vi "MPU_Stick_Queues_FGV.vi"(8 "error in (no error)":errorcluster, 11 "Initialize ?":bool) -> (0 "error out":errorcluster, 3 "MPU_Stick_Queues":T1)   [LabVIEW 2017]
uses:
  Controls/MPU_Stick_Queues.ctl
  Controls/MPU_Stick_Queue_Element.ctl
  Controls/MPU_Stick_Queue_Commands.ctl
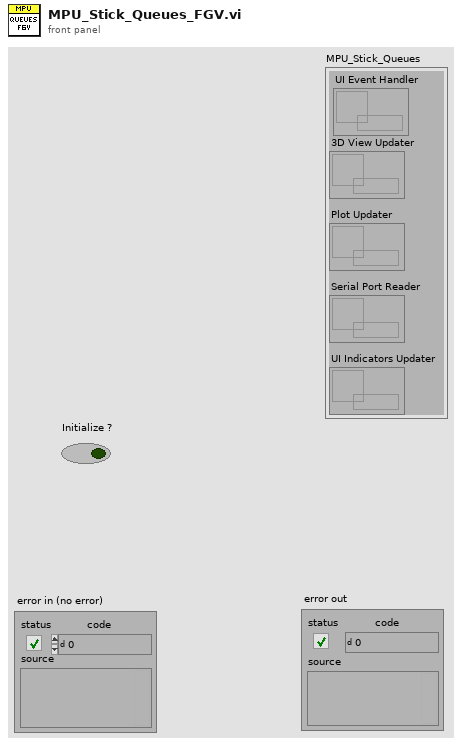
[diagram p1: front panel]
types:
  T1 = typedef "MPU_Stick_Queues.ctl" = cluster{"UI Event Handler":refnum<queue>, "3D View Updater":refnum<queue>, "Plot Updater":refnum<queue>, "Serial Port Reader":refnum<queue>, "UI Indicators Updater":refnum<queue>}
  T2 = typedef "MPU_Stick_Queue_Element.ctl" = cluster{"Data":variant, "Command":T3}
  T3 = typedef "MPU_Stick_Queue_Commands.ctl" = enum16{"UI_Event_Exit_Application_RQST", "UI_Event_Exit_Application_ACK", "UI_Event_Connect_Device_RQST", "UI_Event_Connect_Device_ACK", "UI_Event_Disconnect_Device_RQST", "UI_Event_Disconnect_Device_ACK", "UI_Event_Read_All_Configurations_RQST", "UI_Event_Read_All_Configurations_ACK", "UI_Event_Write_All_Configurations_RQST", "UI_Event_Write_All_Configurations_ACK", "UI_Event_Save_All_Configurations_RQST", "UI_Event_Save_All_Configurations_ACK", "UI_Event_Calibrate_IMU_Sensor_RQST", "UI_Event_Calibrate_IMU_Sensor_ACK", "UI_Event_MP_Reset_RQST", "UI_Event_MP_Reset_ACK", "UI_Event_Get_Config_RQST", "UI_Event_Get_Config_ACK", "UI_Event_Set_Config_RQST", "UI_Event_Set_Config_ACK", "Read_Serial_Port_Data_Pause", "Read_Serial_Port_Data_Continue", "Read_Serial_Port_Data_Exit", "Plotter_Exit", "Plotter_Update", "Plotter_Add_Channel", "Plotter_Remove_Channel", "3D Viewer Update", "3D Viewer Exit", "UI Indicators Update", "UI Indicators Exit"}
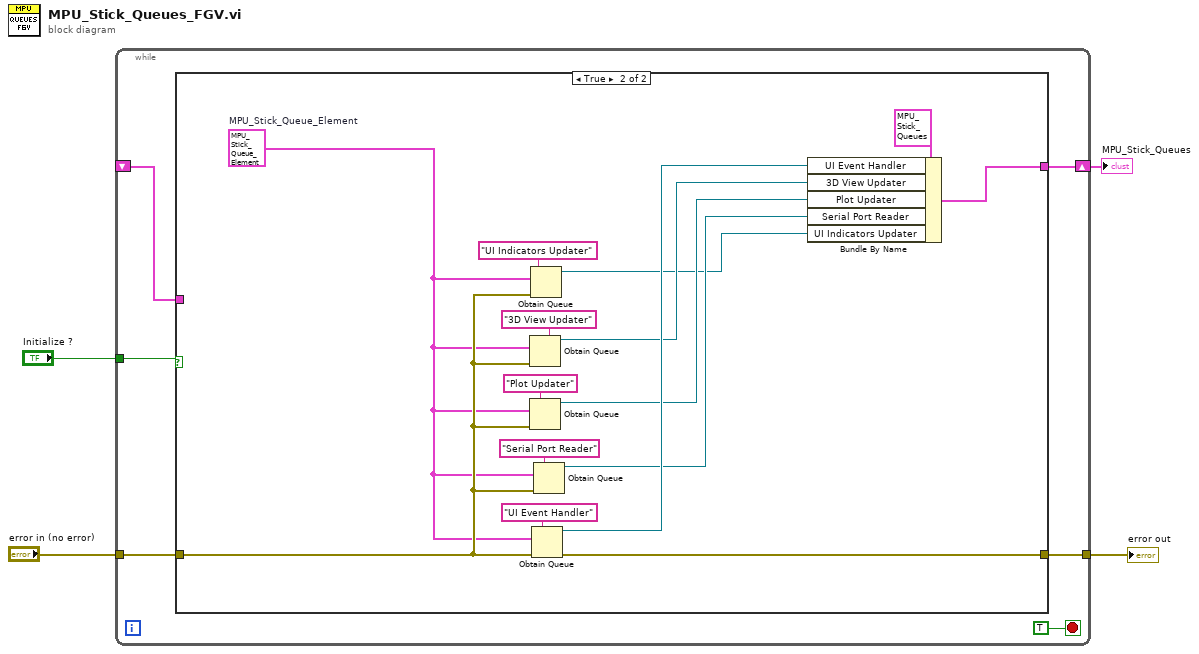
[diagram p0: block diagram]
diagram:
  n1 = while {
    tunnel: "error in (no error)" -> [w9]
    tunnel: [w8] -> w3
    shift-right: [w7] -> w2
    shift-left: _ -> [w6]
    tunnel: "Initialize ?" -> [w5]
    stop <- TRUE stop-if-true
    n2 = case shown="True" w5 {
      tunnel: w9 -> [w11 w15]
      tunnel: [w11 w27] -> w8
      tunnel: [w12 w23] -> w7
      tunnel: w6 -> [w12 _]
      frame False {
      }
      frame True {
        w13 = T2 {"Data"=variant, "Command"=enum."UI_Event_Exit_Application_RQST"}  # MPU_Stick_Queue_Element
        n3 = Obtain Queue(name (unnamed)="3D View Updater", element data type=w13, error in (no error)=w15) -> (queue out=w19:refnum<queue>)  [unwired: 2 in, 2 out]
        n4 = Obtain Queue(name (unnamed)="Plot Updater", element data type=w13, error in (no error)=w15) -> (queue out=w18:refnum<queue>)  [unwired: 2 in, 2 out]
        n5 = Obtain Queue(name (unnamed)="UI Indicators Updater", element data type=w13, error in (no error)=w15) -> (queue out=w14:refnum<queue>)  [unwired: 2 in, 2 out]
        n6 = Obtain Queue(name (unnamed)="UI Event Handler", element data type=w13, error in (no error)=w15) -> (queue out=w24:refnum<queue>, error out=w27:errorcluster)  [unwired: 2 in, 1 out]
        n7 = Obtain Queue(name (unnamed)="Serial Port Reader", element data type=w13, error in (no error)=w15) -> (queue out=w17:refnum<queue>)  [unwired: 2 in, 2 out]
        n8 = Bundle By Name(cluster=T1 {"UI Event Handler"=refnum, "3D View Updater"=refnum, "Plot Updater"=refnum, "Serial Port Reader"=refnum, "UI Indicators Updater"=refnum} ("MPU_Stick_Queues"), "UI Event Handler"=w24, "3D View Updater"=w19, "Plot Updater"=w18, "Serial Port Reader"=w17, "UI Indicators Updater"=w14) -> (w23:T1)
      }
    }
  }
  "error out" <- w3
  "MPU_Stick_Queues" <- w2
